vi "Data Buffering.vi"(10 "Signal":waveform(dbl), 11 "Data in":T1={"First Time"=FALSE, "Show Waterfall Button Clicked"=FALSE, "Data to Process"=0.0, "Slice"=0.0, "window"=1, "averaging parameters"={"averaging mode"=enum."No averaging", "weighting mode"=enum."Exponential", "number of averages"=10}, "Waterfall VI Ref"=refnum, "Signal"={"t0"=timestamp(0 s since 1904-01-01), "dt"=0.0, "Y"=[]}} {"averaging parameters"."number of averages" min=1; "window" items=["Rectangle"=0, "Hanning"=1, "Hamming"=2, "Blackman-Harris"=3, "Exact Blackman"=4, "Blackman"=5, "Flat Top"=6, "4 Term B-Harris "=7, "7 Term B-Harris"=8, "Low Sidelobe"=9, "Blackman Nuttall"=11, "Triangle"=30, "Bartlett-Hanning"=31, "Bohman"=32, "Parzen"=33, "Welch"=34, "Kaiser"=60, "Dolph-Chebyshev"=61, "Gaussian"=62]}) -> (1 "Data Ready":bool, 2 "Data to Process":waveform(dbl), 3 "Data out":T1={"First Time"=FALSE, "Show Waterfall Button Clicked"=FALSE, "Data to Process"=0.0, "Slice"=0.0, "window"=1, "averaging parameters"={"averaging mode"=enum."No averaging", "weighting mode"=enum."Exponential", "number of averages"=10}, "Waterfall VI Ref"=refnum, "Signal"={"t0"=timestamp(0 s since 1904-01-01), "dt"=0.0, "Y"=[]}} {"averaging parameters"."number of averages" min=1; "window" items=["Rectangle"=0, "Hanning"=1, "Hamming"=2, "Blackman-Harris"=3, "Exact Blackman"=4, "Blackman"=5, "Flat Top"=6, "4 Term B-Harris "=7, "7 Term B-Harris"=8, "Low Sidelobe"=9, "Blackman Nuttall"=11, "Triangle"=30, "Bartlett-Hanning"=31, "Bohman"=32, "Parzen"=33, "Welch"=34, "Kaiser"=60, "Dolph-Chebyshev"=61, "Gaussian"=62]})   [LabVIEW 2024, in "Waterfall.lvlib" / "Waterfall.lvclass"]
uses:
  Waterfall.lvclass
  Waterfall Data.ctl
  <vilib>/Analysis/4window.llb/windowTd.ctl
  <vilib>/Analysis/NI_AALPro.lvlib
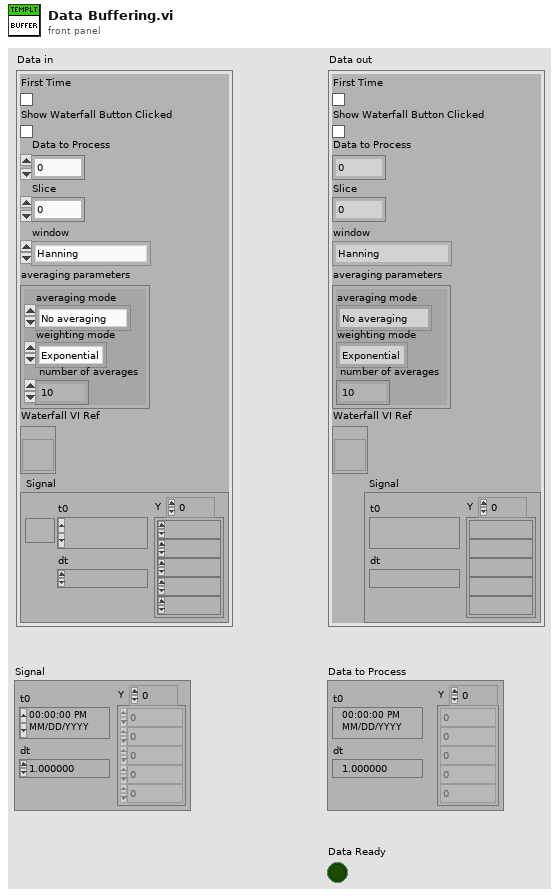
[diagram p1: front panel]
types:
  T1 = typedef "Waterfall.lvlib/Waterfall.lvclass/Waterfall Data.ctl" = cluster{"First Time":bool, "Show Waterfall Button Clicked":bool, "Data to Process":dbl, "Slice":dbl, "window":T2, "averaging parameters":cluster{"averaging mode":enum16{"No averaging", "Vector averaging", "RMS averaging", "Peak hold"}, "weighting mode":enum16{"Linear", "Exponential"}, "number of averages":u32}, "Waterfall VI Ref":refnum<vi>, "Signal":waveform(dbl)}
  T2 = typedef "NI_AALPro.lvlib/windowTd.ctl" = u32
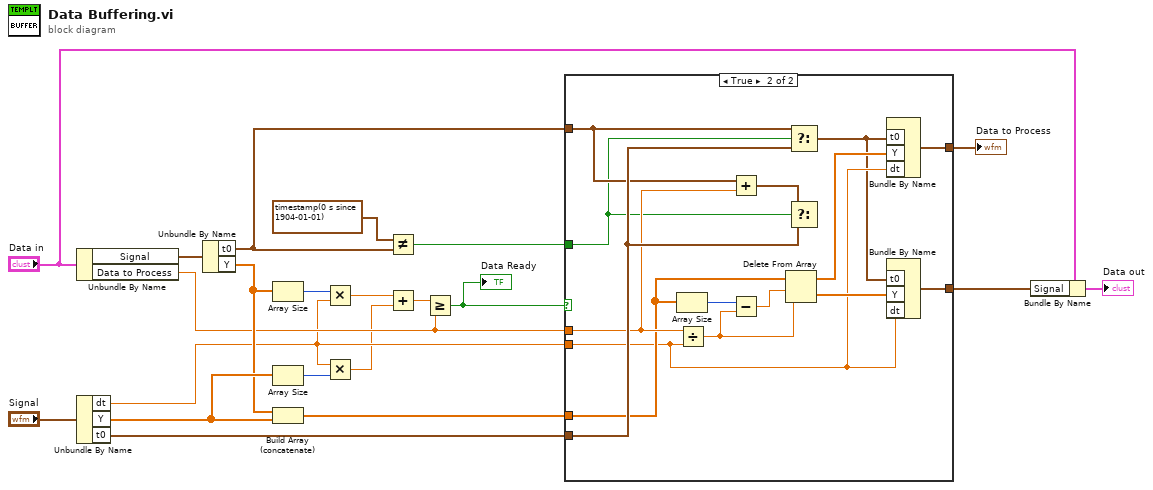
[diagram p0: block diagram]
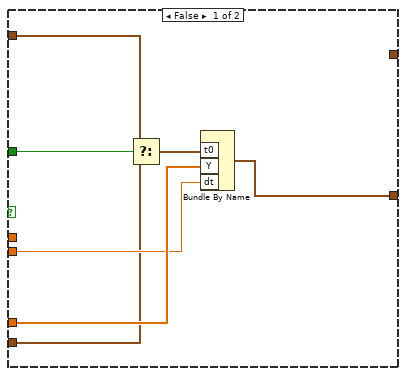
[diagram p2: hidden frame]
diagram:
  n1 = Unbundle By Name("Data in") -> ("Signal"=w20:waveform(dbl), "Data to Process"=w13:dbl)
  n2 = Unbundle By Name("Signal") -> ("dt"=w6:dbl, "Y"=w16:dbl[], "t0"=w12:timestamp)
  n3 = Unbundle By Name(w20) -> ("t0"=w8:timestamp, "Y"=w15:dbl[])
  n4 = Array Size(array=w15) -> (size(s)=w19:i32)
  n5 = Array Size(array=w16) -> (size(s)=w18:i32)
  n6 = Build Array (concatenate)(w15, w16) -> (w14:dbl[])
  n7 = Multiply(x=w19, y=w6) -> (x*y=w5:dbl)
  n8 = Multiply(x=w6, y=w18) -> (x*y=w4:dbl)
  n9 = Not Equal?(x=timestamp(0 s since 1904-01-01) ("y"), y=w8) -> (x != y?=w7:bool)
  n10 = Add(x=w5, y=w4) -> (x+y=w17:dbl)
  n11 = Greater Or Equal?(x=w17, y=w13) -> (x >= y?=w3:bool)
  "Data Ready" <- w3
  n12 = case shown="True" w3 {
    tunnel: w14 -> [w27 w38]
    tunnel: w13 -> [_ w39]
    tunnel: w6 -> [w26 w33]
    tunnel: w8 -> [w24 w31]
    tunnel: w12 -> [w23 w42]
    tunnel: [_ w43] -> w11
    tunnel: [w22 w32] -> w10
    tunnel: w7 -> [w25 w30]
    frame False {
      n13 = Select(t=w24, s=w25, f=w23) -> (s? t:f=w28:timestamp)
      n14 = Bundle By Name("t0"=w28, "Y"=w27, "dt"=w26) -> (w22:waveform(dbl))  [unwired: 1 in]
    }
    frame True {
      n15 = Array Size(array=w38) -> (size(s)=w37:i32)
      n16 = Divide(x=w39, y=w33) -> (x/y=w36:dbl)
      n17 = Add(x=w31, y=w39) -> (x+y=w41:timestamp)
      n18 = Subtract(x=w37, y=w36) -> (x-y=w35:dbl)
      n19 = Delete From Array(array=w38, length=w35, index=w36) -> (deleted portion=w34:dbl[], array with subset deleted=w40:dbl[])
      n20 = Select(t=w31, s=w30, f=w42) -> (s? t:f=w29:timestamp)
      n21 = Select(t=w41, s=w30, f=w42) -> ()  [unwired: 1 out]
      n22 = Bundle By Name("t0"=w29, "Y"=w40, "dt"=w33) -> (w43:waveform(dbl))  [unwired: 1 in]
      n23 = Bundle By Name("t0"=w29, "Y"=w34, "dt"=w33) -> (w32:waveform(dbl))  [unwired: 1 in]
    }
  }
  "Data to Process" <- w11
  n24 = Bundle By Name(cluster="Data in", "Signal"=w10) -> (→"Data out":T1)
